vi "VIPM_Build Internal Target Map.vi"(11 "Package Array":T1[](array[typedef])) -> (3 "Internal Target Map":map{string, string}(c390))   [LabVIEW 2019]
doc: "Build an 'Internal Target Map' from the given 'Package Array'"
uses:
  Ctl/Ctl_Package Identifier Cluster.ctl
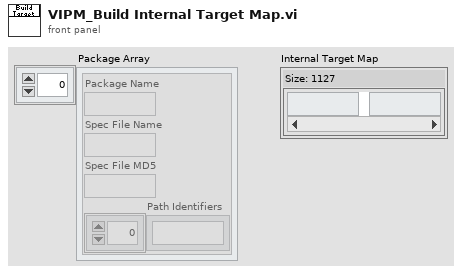
[diagram p1: front panel]
types:
  T1 = typedef "Ctl_Package Identifier Cluster.ctl" = cluster{"Package Name":string, "Spec File Name":string, "Spec File MD5":string, "Path Identifiers":string[]}
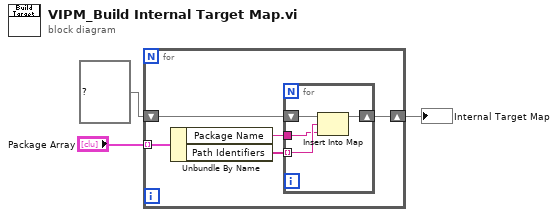
[diagram p0: block diagram]
diagram:
  n1 = for {
    tunnel: "Package Array" -> [w8] mode=indexing
    shift-right: [w6] -> w3
    shift-left: map{string, string} {} ("Internal Target Map") -> [w7]
    n2 = Unbundle By Name(w8) -> ("Package Name"=w4:string, "Path Identifiers"=w5:string[])
    n3 = for {
      shift-right: [w11] -> w6
      shift-left: w7 -> [w12]
      tunnel: w5 -> [w10] mode=indexing
      tunnel: w4 -> [w9]
      n4 = Insert Into Map(map in=w12, key=w10, value=w9) -> (map out=w11:map{string, string})  [unwired: 2 out]
    }
  }
  "Internal Target Map" <- w3
